vi "encendido de led rgb.vi"() -> ()   [LabVIEW 2016]
uses:
  <vilib>/LabVIEW Interface for Arduino/Type Defs/Board Type.ctl
  <vilib>/LabVIEW Interface for Arduino/Type Defs/Connection Type.ctl
  <vilib>/LabVIEW Interface for Arduino/LabVIEW Interface for Arduino.lvlib
panel:
  out "Color":u32(colorbox)
  in  "Stop Button":bool
  in  "BLUE":u32(knob) scale=0.0..255.0
  in  "GREEN":u32(knob) scale=0.0..255.0
  in  "RED":u32(knob) scale=0.0..255.0
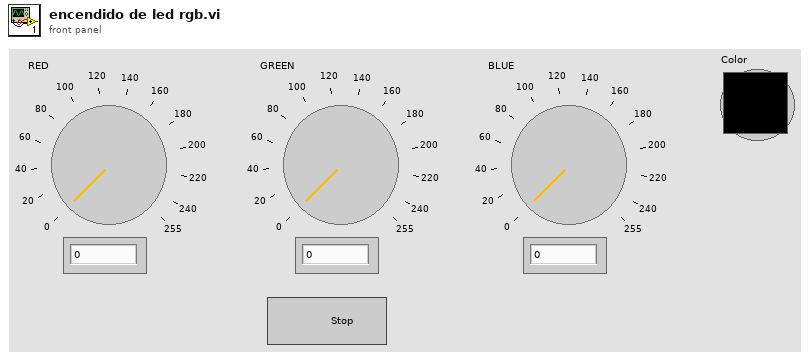
[diagram p1: front panel]
types:
  T1 = typedef "LabVIEW Interface for Arduino.lvlib/Connection Type.ctl" = enum8{"USB / Serial", "XBEE", "BlueSmirf (Bluetooth)"}
  T2 = typedef "LabVIEW Interface for Arduino.lvlib/Board Type.ctl" = enum16{"Uno", "Dimuelanove w/Atmega 328", "Mega 2560"}
  T3 = typedef "LabVIEW Interface for Arduino.lvlib/Arduino Resource.ctl" = cluster{"VISA resource":refnum<visa-resource-name>, "Board Type":T2, "Connection Type":enum8{"USB / Serial"}, "Bytes Per Packet (15)":u8}
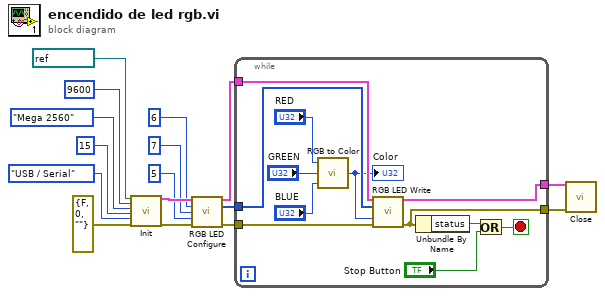
[diagram p0: block diagram]
diagram:
  n1 = call <vilib>:"Init.vi"("VISA resource"=refnum<visa-resource-name> "COM6", "Baud Rate (115200)"=u32 9600, "Board Type (Uno)"=Board_Type."Mega 2560", "Bytes Per Packet (15)"=u32 15, "Connection Type (USB/Serial)"=Connection_Type."USB / Serial", "error in"=errorcluster {"status"=FALSE, "code"=0, "source"=""}) -> ("Arduino Resource"=w10:T3, "error out"=w9:errorcluster)  [unwired: 12 in]
  n2 = call <vilib>:"RGB LED Configure.vi"("Arduino Resource"=w10, "Red Pin"=u8 6, "Green Pin"=u8 7, "Blue Pin"=u8 5, "error in"=w9) -> ("Arduino Resource"=w5:T3, "RGB LED Pins"=w3:u8[], "error out"=w4:errorcluster)  [unwired: 8 in]
  n3 = while {
    tunnel: w5 -> [w28]
    tunnel: w4 -> [w27]
    tunnel: w3 -> [w26]
    tunnel: [w18] -> w2
    tunnel: [w17] -> w1
    stop <- w20 stop-if-true
    n4 = call <vilib>:"RGB to Color.vi"("B"="BLUE", "G"="GREEN", "R"="RED") -> ("Color"=w22:u32)
    "Color" <- w22
    n5 = call <vilib>:"RGB LED Write.vi"("Arduino Resource"=w28, "RGB LED Pins"=w26, "Color"=w22, "error in"=w27) -> ("Arduino Resource"=w18:T3, "error out"=w17:errorcluster)  [unwired: 9 in, 1 out]
    n6 = Unbundle By Name(w17) -> ("status"=w21:bool)
    n7 = Or(x=w21, y="Stop Button") -> (x .or. y?=w20:bool)
  }
  n8 = call <vilib>:"Close.vi"("Arduino Resource"=w2, "error in"=w1) -> ()  [unwired: 13 in, 1 out]
